vi "Obtain Request Events.vi"(8 "error in":errorcluster, 10 "Create New? (F)":bool) -> (0 "error out":errorcluster, 2 "Acquisition Request Events":T1)   [LabVIEW 2020, in "Acquisition.lvlib"]
doc: "This VI Obtains/Creates the Requests events that will be used for other modules to communicate with the module that owns this VI. These Requests events will be accessed only via Public API methods for this module.\n\n<b>NOTE</b>: The contents of this VI are automatically generated and modified by the <b>Tools > DQMH Consortium > DQMH</b> utilities. Consider using those utilities instead of making your own modifications to this VI.\n_____\nBased on DQMH Project Template 4.0.0.47.\n_____\nBased on DQMH Project Template 7.0.1.1316."
uses:
  Acquisition.lvlib
  Request Events--cluster.ctl
  Stop Argument--cluster.ctl
  Show Panel Argument--cluster.ctl
  Hide Panel Argument--cluster.ctl
  Get Module Execution Status Argument--cluster.ctl
  Show Diagram Argument--cluster.ctl
  Stop Acquiring Argument--cluster.ctl
  Wakeup Helper Loop Argument--cluster.ctl
  Change Settings Argument--cluster.ctl
  CML Shared/Signal Type--enum.ctl
  CML Shared/Calibration Values--cluster.ctl
  Calibrate DAQ Argument--cluster.ctl
  Start Acquiring Argument--cluster.ctl
  Start Acquiring (Reply Payload)--cluster.ctl
  CML Shared/CML Shared.lvlib
panel:
  # "NOTE: The contents of this VI are automatically generated and modified by the Tools > DQMH Consortium > DQMH utilities. Consider using those utilities instead of making your own modifications to this VI."
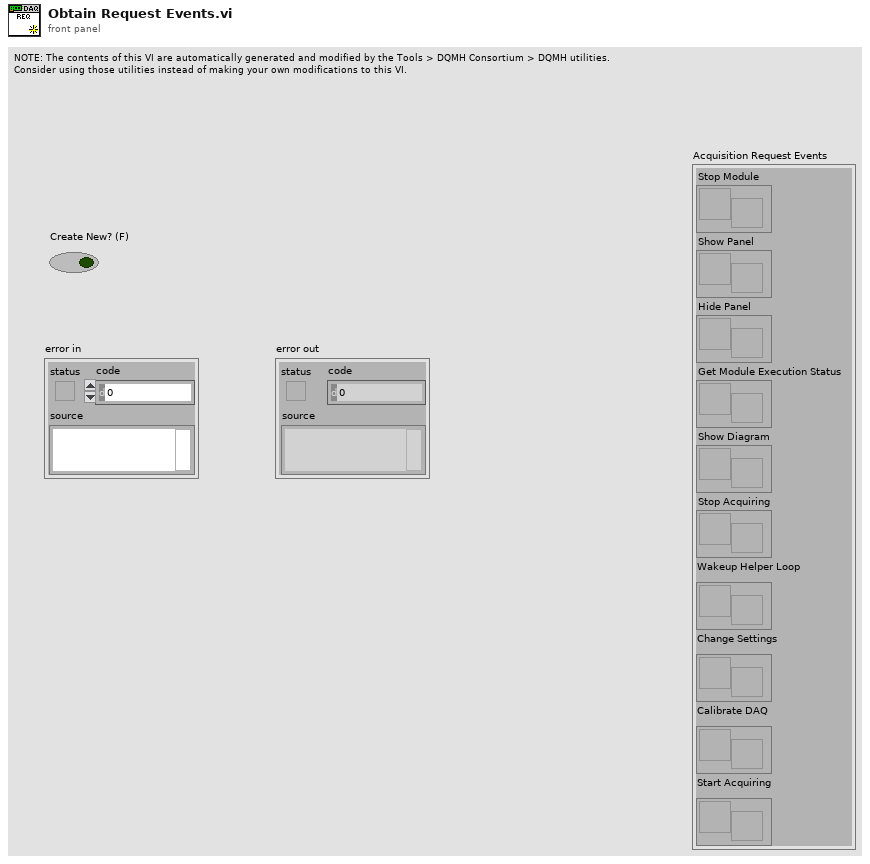
[diagram p1: front panel]
types:
  T1 = typedef "Acquisition.lvlib/Request Events--cluster.ctl" = cluster{"Stop Module":refnum<user-event>, "Show Panel":refnum<user-event>, "Hide Panel":refnum<user-event>, "Get Module Execution Status":refnum<user-event>, "Show Diagram":refnum<user-event>, "Stop Acquiring":refnum<user-event>, "Wakeup Helper Loop":refnum<user-event>, "Change Settings":refnum<user-event>, "Calibrate DAQ":refnum<user-event>, "Start Acquiring":refnum<user-event>}
  T2 = typedef "Acquisition.lvlib/Start Acquiring Argument--cluster.ctl" = cluster{"Wait Notifier":refnum<notifier>, "wait for reply":bool}
  T3 = typedef "Acquisition.lvlib/Calibrate DAQ Argument--cluster.ctl" = cluster{"None":bool}
  T4 = typedef "Acquisition.lvlib/Change Settings Argument--cluster.ctl" = cluster{"Signal Type":T5, "Calibration Array":T6[]}
  T5 = typedef "CML Shared.lvlib/Signal Type--enum.ctl" = enum16{"Sine Wave", "Square with Noise"}
  T6 = typedef "CML Shared.lvlib/Calibration Values--cluster.ctl" = cluster{"Slope":dbl, "Offset":dbl}
  T7 = typedef "Acquisition.lvlib/Wakeup Helper Loop Argument--cluster.ctl" = cluster{"HW ID":string}
  T8 = typedef "Acquisition.lvlib/Stop Acquiring Argument--cluster.ctl" = cluster{"Boolean":bool}
  T9 = typedef "Acquisition.lvlib/Hide Panel Argument--cluster.ctl" = cluster{"Hide Panel?":bool}
  T10 = typedef "Acquisition.lvlib/Show Panel Argument--cluster.ctl" = cluster{"Show Panel?":bool}
  T11 = typedef "Acquisition.lvlib/Show Diagram Argument--cluster.ctl" = cluster{"Debug?":bool}
  T12 = typedef "Acquisition.lvlib/Get Module Execution Status Argument--cluster.ctl" = cluster{"Running?":bool}
  T13 = typedef "Acquisition.lvlib/Stop Argument--cluster.ctl" = cluster{"Origin":string, "Exit via Stop Module Req?":bool, "Wait for Module to stop?":bool}
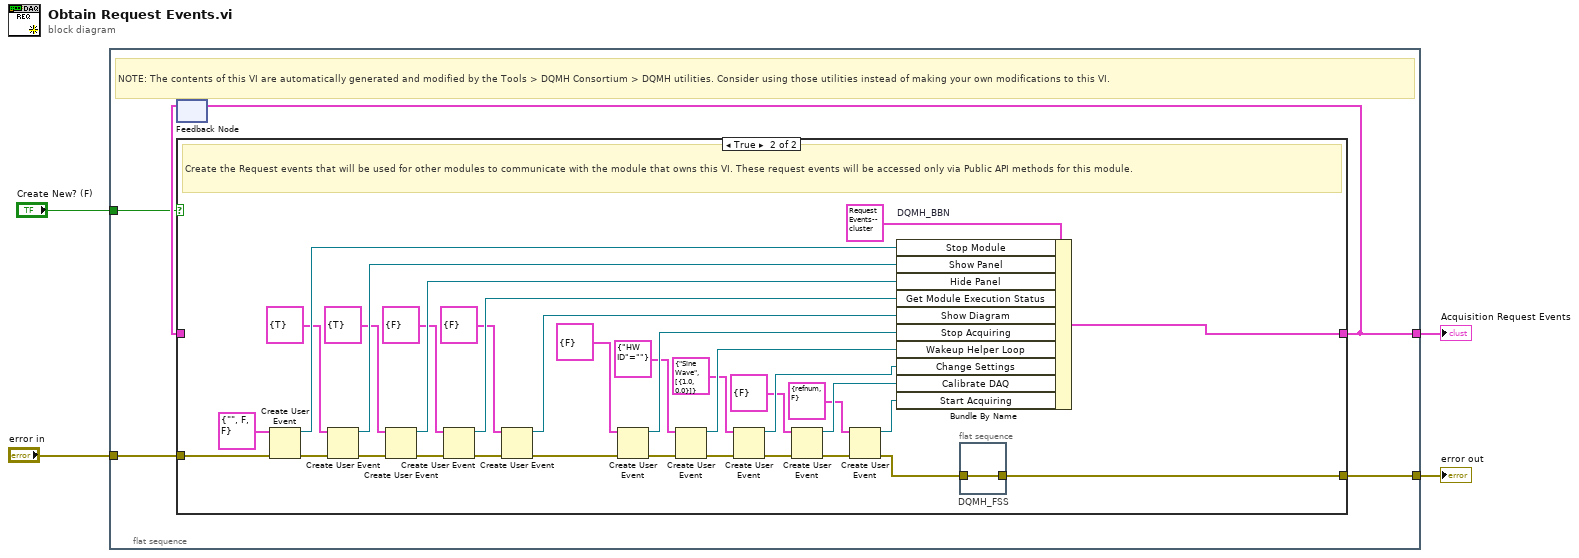
[diagram p0: block diagram]
diagram:
  n1 = flat-sequence {
    tunnel: [w9] -> w4
    tunnel: "error in" -> [w8]
    tunnel: [w6] -> w2
    tunnel: "Create New? (F)" -> [w5]
    frame #0 {
      # "NOTE: The contents of this VI are automatically generated and modified by the Tools > DQMH Consortium > DQMH utilities. Consider using those utilities instead of making your own modifications to this VI."
      n2 = feedback #1() -> (w7:T1)  [unwired: 1 in]
      n3 = case shown="True" w5 {
        tunnel: [w10 w35] -> w9
        tunnel: w8 -> [w10 w45]
        tunnel: [w11 w42] -> w6
        tunnel: w7 -> [w11 _]
        frame False {
          # "Obtain the Request events that were created in a previous call to this VI."
        }
        frame True {
          # "Create the Request events that will be used for other modules to communicate with the module that owns this VI. These request events will be accessed only via Public API methods for this module."
          n4 = Create User Event(user event datatype=T13 {"Origin"="", "Exit via Stop Module Req?"=FALSE, "Wait for Module to stop?"=FALSE} ("Stop Argument"), error in=w45) -> (user event=w43:refnum<user-event>, error out=w40:errorcluster)
          n5 = Create User Event(user event datatype=T10 {"Show Panel?"=TRUE} ("Show Panel Argument"), error in=w40) -> (user event=w39:refnum<user-event>, error out=w38:errorcluster)
          n6 = Create User Event(user event datatype=T9 {"Hide Panel?"=TRUE} ("Hide Panel Argument"), error in=w38) -> (user event=w37:refnum<user-event>, error out=w36:errorcluster)
          n7 = Create User Event(user event datatype=T12 {"Running?"=FALSE} ("Get Module Execution Status Argument"), error in=w36) -> (user event=w33:refnum<user-event>, error out=w34:errorcluster)
          n8 = Create User Event(user event datatype=T11 {"Debug?"=FALSE} ("Show Diagram Argument"), error in=w34) -> (user event=w30:refnum<user-event>, error out=w31:errorcluster)
          n9 = Create User Event(user event datatype=T8 {"Boolean"=FALSE} ("Stop Acquiring Argument"), error in=w31) -> (user event=w25:refnum<user-event>, error out=w26:errorcluster)
          n10 = Create User Event(user event datatype=T7 {"HW ID"=""} ("Wakeup Message Pump Argument"), error in=w26) -> (user event=w22:refnum<user-event>, error out=w23:errorcluster)
          n11 = Create User Event(user event datatype=T4 {"Signal Type"=enum."Sine Wave", "Calibration Array"=[{"Slope"=1.0, "Offset"=0.0}]} ("Change Settings Argument"), error in=w23) -> (user event=w19:refnum<user-event>, error out=w20:errorcluster)
          n12 = Create User Event(user event datatype=T3 {"None"=FALSE} ("Calibrate DAQ Argument"), error in=w20) -> (user event=w16:refnum<user-event>, error out=w17:errorcluster)
          n13 = Create User Event(user event datatype=T2 {"Wait Notifier"=refnum, "wait for reply"=FALSE} ("Start Acquisition Argument"), error in=w17) -> (user event=w13:refnum<user-event>, error out=w14:errorcluster)
          n14 = Bundle By Name "DQMH_BBN"(cluster=T1 {"Stop Module"=refnum, "Show Panel"=refnum, "Hide Panel"=refnum, "Get Module Execution Status"=refnum, "Show Diagram"=refnum, "Stop Acquiring"=refnum, "Wakeup Helper Loop"=refnum, "Change Settings"=refnum, "Calibrate DAQ"=refnum, "Start Acquiring"=refnum} ("output cluster"), "Stop Module"=w43, "Show Panel"=w39, "Hide Panel"=w37, "Get Module Execution Status"=w33, "Show Diagram"=w30, "Stop Acquiring"=w25, "Wakeup Helper Loop"=w22, "Change Settings"=w19, "Calibrate DAQ"=w16, "Start Acquiring"=w13) -> (w42:T1)
          n15 = flat-sequence "DQMH_FSS" {
            tunnel: w14 -> [w46]
            tunnel: [w46] -> w35
            frame #0 {
            }
          }
        }
      }
      n16 = feedback-in #1(w6) -> ()
    }
  }
  "Acquisition Request Events" <- w2
  "error out" <- w4
